vi "Write Image.vi"(8 "error in (no error)":errorcluster, 10 "Matrix":T1[][](array[typedef]) items=["red"=0, "orange"=18, "yellow"=24, "green"=82, "cyan"=127, "blue"=170, "purple"=195, "pink"=220, "white"=254, "black"=255], 11 "Grove 2 RGB LED Matrix In":refnum<class "Grove 2 RGB LED Matrix.lvclass">) -> (0 "error out":errorcluster, 3 "Grove 2 RGB LED Matrix Out":refnum<class "Grove 2 RGB LED Matrix.lvclass">)   [LabVIEW 2020, in "CTI-Peripheral.lvlib" / "Grove 2 RGB LED Matrix.lvclass"]
uses:
  Grove 2 RGB LED Matrix.lvclass
  Data Types/Colors.ctl
  Data Types/MatrixI2CCommand.ctl
  Grove 2 RGB LED Matrix.lvclass/Grove 2 RGB LED Matrix.ctl
  CTI/I2C Connection/I2C Connection.lvclass/I2C Connection.ctl
  CTI/Session/I2C Write Data.vi
  CTI/I2C Connection/I2C Connection.lvclass
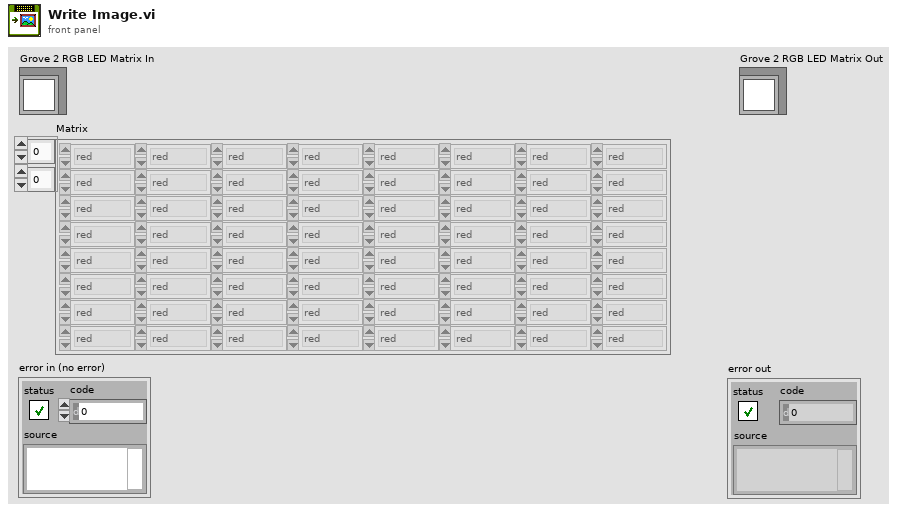
[diagram p1: front panel]
types:
  T1 = typedef "CTI-Peripheral.lvlib/Grove 2 RGB LED Matrix.lvclass/Colors.ctl" = u8
  T2 = typedef "CTI-Peripheral.lvlib/Grove 2 RGB LED Matrix.lvclass/MatrixI2CCommand.ctl" = u8
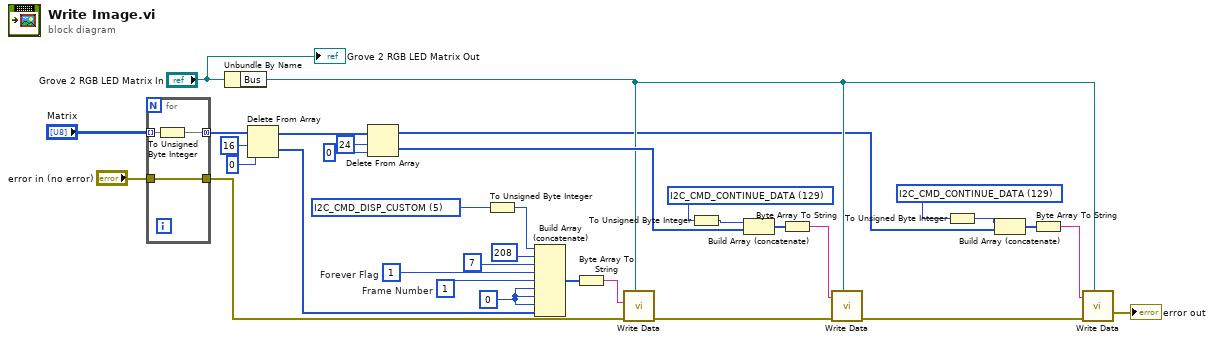
[diagram p0: block diagram]
diagram:
  w2 = u8 1  # Frame Number
  w5 = T2 129 items=["I2C_CMD_GET_DEV_ID"=0, "I2C_CMD_DISP_BAR"=1, "I2C_CMD_DISP_EMOJI"=2, "I2C_CMD_DISP_NUM"=3, "I2C_CMD_DISP_STR"=4, "I2C_CMD_DISP_CUSTOM"=5, "I2C_CMD_DISP_OFF"=6, "I2C_CMD_DISP_ASCII"=7, "I2C_CMD_DISP_FLASH"=8, "I2C_CMD_DISP_COLOR_BAR"=9, "I2C_CMD_DISP_COLOR_WAVE"=10, "I2C_CMD_DISP_COLOR_CLOCKWISE"=11, "I2C_CMD_DISP_COLOR_ANIMATION"=12, "I2C_CMD_DISP_COLOR_BLOCK "=13, "I2C_CMD_CONTINUE_DATA"=129, "I2C_CMD_STORE_FLASH"=160, "I2C_CMD_DELETE_FLASH"=161, "I2C_CMD_LED_ON"=176, "I2C_CMD_LED_OFF"=177, "I2C_CMD_AUTO_SLEEP_ON"=178, "I2C_CMD_AUTO_SLEEP_OFF"=179, "I2C_CMD_DISP_ROTATE"=180, "I2C_CMD_DISP_OFFSET"=181, "I2C_CMD_SET_ADDR"=192, "I2C_CMD_RST_ADDR"=193, "I2C_CMD_TEST_GET_VER"=226, "I2C_CMD_GET_DEVICE_UID"=241] ("I2C Command")
  w3 = u8 0 ("Forever Flag")
  w25 = u8 1  # Forever Flag
  w9 = T2 5 items=["I2C_CMD_GET_DEV_ID"=0, "I2C_CMD_DISP_BAR"=1, "I2C_CMD_DISP_EMOJI"=2, "I2C_CMD_DISP_NUM"=3, "I2C_CMD_DISP_STR"=4, "I2C_CMD_DISP_CUSTOM"=5, "I2C_CMD_DISP_OFF"=6, "I2C_CMD_DISP_ASCII"=7, "I2C_CMD_DISP_FLASH"=8, "I2C_CMD_DISP_COLOR_BAR"=9, "I2C_CMD_DISP_COLOR_WAVE"=10, "I2C_CMD_DISP_COLOR_CLOCKWISE"=11, "I2C_CMD_DISP_COLOR_ANIMATION"=12, "I2C_CMD_DISP_COLOR_BLOCK "=13, "I2C_CMD_CONTINUE_DATA"=129, "I2C_CMD_STORE_FLASH"=160, "I2C_CMD_DELETE_FLASH"=161, "I2C_CMD_LED_ON"=176, "I2C_CMD_LED_OFF"=177, "I2C_CMD_AUTO_SLEEP_ON"=178, "I2C_CMD_AUTO_SLEEP_OFF"=179, "I2C_CMD_DISP_ROTATE"=180, "I2C_CMD_DISP_OFFSET"=181, "I2C_CMD_SET_ADDR"=192, "I2C_CMD_RST_ADDR"=193, "I2C_CMD_TEST_GET_VER"=226, "I2C_CMD_GET_DEVICE_UID"=241] ("I2C Command")
  w7 = T2 129 items=["I2C_CMD_GET_DEV_ID"=0, "I2C_CMD_DISP_BAR"=1, "I2C_CMD_DISP_EMOJI"=2, "I2C_CMD_DISP_NUM"=3, "I2C_CMD_DISP_STR"=4, "I2C_CMD_DISP_CUSTOM"=5, "I2C_CMD_DISP_OFF"=6, "I2C_CMD_DISP_ASCII"=7, "I2C_CMD_DISP_FLASH"=8, "I2C_CMD_DISP_COLOR_BAR"=9, "I2C_CMD_DISP_COLOR_WAVE"=10, "I2C_CMD_DISP_COLOR_CLOCKWISE"=11, "I2C_CMD_DISP_COLOR_ANIMATION"=12, "I2C_CMD_DISP_COLOR_BLOCK "=13, "I2C_CMD_CONTINUE_DATA"=129, "I2C_CMD_STORE_FLASH"=160, "I2C_CMD_DELETE_FLASH"=161, "I2C_CMD_LED_ON"=176, "I2C_CMD_LED_OFF"=177, "I2C_CMD_AUTO_SLEEP_ON"=178, "I2C_CMD_AUTO_SLEEP_OFF"=179, "I2C_CMD_DISP_ROTATE"=180, "I2C_CMD_DISP_OFFSET"=181, "I2C_CMD_SET_ADDR"=192, "I2C_CMD_RST_ADDR"=193, "I2C_CMD_TEST_GET_VER"=226, "I2C_CMD_GET_DEVICE_UID"=241] ("I2C Command")
  n1 = for {
    tunnel: "error in (no error)" -> [w37]
    tunnel: [w37] -> w23
    tunnel: "Matrix" -> [w36] mode=indexing
    tunnel: [w35] -> w30 mode=concatenating
    n2 = To Unsigned Byte Integer(number=w36) -> (unsigned 8bit integer=w35:T1[])
  }
  n3 = Unbundle By Name("Grove 2 RGB LED Matrix In") -> ("Bus"=w11:refnum<class "I2C Connection.lvclass">)
  n4 = Delete From Array(array=w30, length=16, index=0) -> (deleted portion=w24:T1[], array with subset deleted=w21:T1[])
  n5 = Delete From Array(array=w21, length=24, index=0) -> (deleted portion=w18:T1[], array with subset deleted=w10:T1[])
  n6 = To Unsigned Byte Integer(number=w9) -> (unsigned 8bit integer=w8:T2)
  n7 = Build Array (concatenate)(w8, u8 208, u8 7, w25, w2, w3, w3, w3, w24) -> (w32:T1[])
  n8 = Byte Array To String(unsigned byte array=w32) -> (string=w31:string)
  n9 = call "Write Data.vi"("I2C Connection"=w11, "error in (no error)"=w23, "Data"=w31) -> ("error out"=w16:errorcluster)  [unwired: 8 in]
  n10 = To Unsigned Byte Integer(number=w7) -> (unsigned 8bit integer=w6:T2)
  n11 = Build Array (concatenate)(w6, w18) -> (w17:T1[])
  n12 = Byte Array To String(unsigned byte array=w17) -> (string=w22:string)
  n13 = call "Write Data.vi"("I2C Connection"=w11, "error in (no error)"=w16, "Data"=w22) -> ("error out"=w12:errorcluster)  [unwired: 8 in]
  n14 = To Unsigned Byte Integer(number=w5) -> (unsigned 8bit integer=w4:T2)
  n15 = Build Array (concatenate)(w4, w10) -> (w15:T1[])
  n16 = Byte Array To String(unsigned byte array=w15) -> (string=w14:string)
  n17 = call "Write Data.vi"("I2C Connection"=w11, "error in (no error)"=w12, "Data"=w14) -> ("error out"=→"error out":errorcluster)  [unwired: 8 in]
  "Grove 2 RGB LED Matrix Out" <- "Grove 2 RGB LED Matrix In"
